vi "Profiles File Key--constant.vi"() -> (3 "Profiles File Key":string="EnvironmentToolkit.ProfilesFile")   [LabVIEW 2025]
doc: "This constant represents the Profiles File Key String in the LabVIEW INI File."
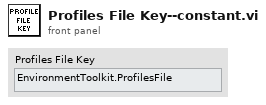
[diagram p1: front panel]
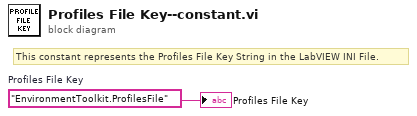
[diagram p0: block diagram]
diagram:
  w1 = "EnvironmentToolkit.ProfilesFile"  # Profiles File Key
  # "This constant represents the Profiles File Key String in the LabVIEW INI File."
  "Profiles File Key" <- w1
